vi "Remove Prefix.vi"(10 "Prefix":string, 11 "String":string) -> (2 "Prefix Missing?":bool, 3 "String out":string)   [LabVIEW 2015, in "E2E Tag Exchange editor node.lvclass"]
uses:
  E2E Tag Exchange editor node.lvclass
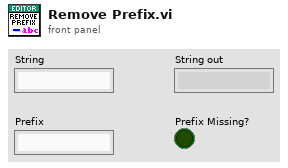
[diagram p1: front panel]
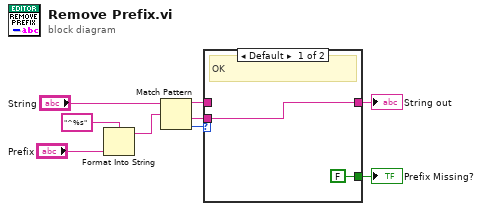
[diagram p0: block diagram]
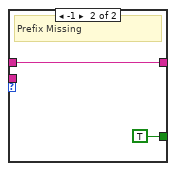
[diagram p2: hidden frame]
diagram:
  n1 = Format Into String(format string="^%s", "Prefix") -> (resulting string=w4:string)  [unwired: 2 in, 1 out]
  n2 = Match Pattern(string="String", regular expression=w4) -> (before substring=w6:string, after substring=w1:string, offset past match=w7:i32)  [unwired: 1 in, 1 out]
  n3 = case shown="Default" w7 {
    tunnel: [FALSE TRUE] -> w9
    tunnel: w6 -> [_ w12]
    tunnel: [w10 w12] -> w2
    tunnel: w1 -> [w10 _]
    frame Default {
      # "OK"
    }
    frame -1 {
      # "Prefix Missing"
    }
  }
  "Prefix Missing?" <- w9
  "String out" <- w2
